vi "DeInit.vi"(8 "error in (no error)":errorcluster, 11 "ZWO_ASI in":refnum<class "ZWO_ASI.lvclass">) -> (0 "error out":errorcluster, 3 "ZWO_ASI out":refnum<class "ZWO_ASI.lvclass">)   [LabVIEW 2023, in "ZWO_ASI.lvlib" / "ZWO_ASI.lvclass"]
uses:
  ZWO_ASI.lvclass
  Labview_ASI_demo_64bit_221128/user.lib/ASICamera2_no_err/ASICamera2_no_err.lvlib
  UIs/InterferometryUI/InterferometryUI Messages/DeInit Done Msg/DeInit Done Msg.lvclass
  <vilib>/ActorFramework/Actor/Actor.lvclass
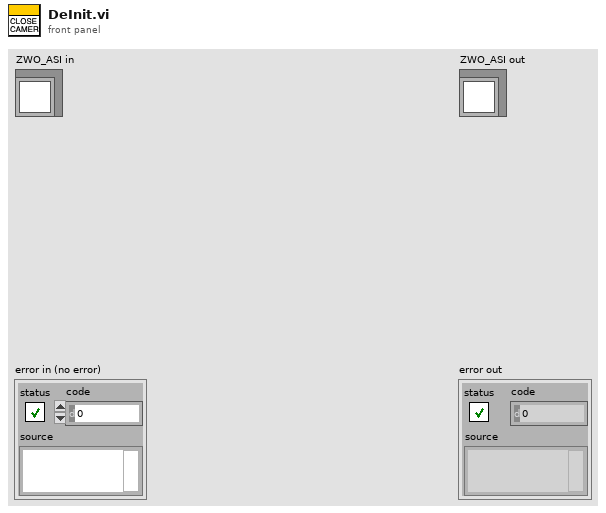
[diagram p1: front panel]
types:
  T1 = typedef "typedefs.lvlib/InstrumentData.ctl" = cluster{"Instr Error":errorcluster, "Address":cluster{"address type":enum16{"VISA", "Index"}, "Address":string, "instrument type":T2}, "CurrentState":cluster{"Initialized":bool, "Connected":bool, "Running":bool, "Error":bool}, "Enqueuer":refnum<class "Message Enqueuer.lvclass">}
  T2 = typedef "typedefs.lvlib/instrumentType.ctl" = enum16{"Spectrometer", "Camera", "Stepper"}
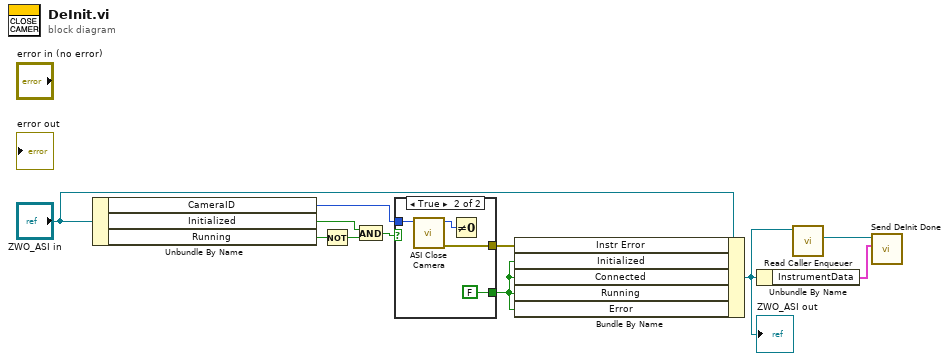
[diagram p0: block diagram]
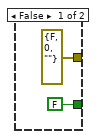
[diagram p2: hidden frame]
diagram:
  n1 = Unbundle By Name("ZWO_ASI in") -> ("CameraID"=w11:i32, "Initialized"=w9:bool, "Running"=w10:bool)
  n2 = Not(x=w10) -> (.not. x?=w8:bool)
  n3 = And(x=w9, y=w8) -> (x .and. y?=w7:bool)
  n4 = case shown="True" w7 {
    tunnel: w11 -> [_ w17]
    tunnel: [errorcluster {"status"=FALSE, "code"=0, "source"=""} ("error out") w15] -> w6
    tunnel: [FALSE FALSE] -> w5
    frame False {
    }
    frame True {
      n5 = call "ASI Close Camera.vi"("iCameraID"=w17) -> ("error out"=w15:errorcluster, "function return"=w16:i32)  [unwired: 9 in]
      n6 = Not Equal To 0?(x=w16) -> ()  [unwired: 1 out]
    }
  }
  n7 = Bundle By Name(cluster="ZWO_ASI in", "Instr Error"=w6, "Initialized"=w5, "Connected"=w5, "Running"=w5, "Error"=w5) -> (w2:refnum<class "ZWO_ASI.lvclass">)
  "ZWO_ASI out" <- w2
  n8 = Unbundle By Name(w2) -> ("InstrumentData"=w1:T1)
  n9 = call <vilib>:"Read Caller Enqueuer.vi"("Actor"=w2) -> ("Caller Enqueuer"=w4:refnum<class "Message Enqueuer.lvclass">)  [unwired: 10 in]
  n10 = call "Send DeInit Done.vi"("InstrumentData"=w1, "Message Enqueuer"=w4) -> ()  [unwired: 8 in, 2 out]
